vi "Estimate Time.vi"(8 "error in (no error)":errorcluster, 11 "Scheduler in":refnum<class "Scheduler.lvclass">) -> (0 "error out":errorcluster, 3 "Scheduler out":refnum<class "Scheduler.lvclass">)   [LabVIEW 2020, in "Scheduler.lvlib" / "Scheduler.lvclass"]
uses:
  Scheduler.lvclass
  Scheduler.lvclass/Scheduler.ctl
  Run Utilities/Sequence of SBlocks/Sequence of SBlocks.lvclass
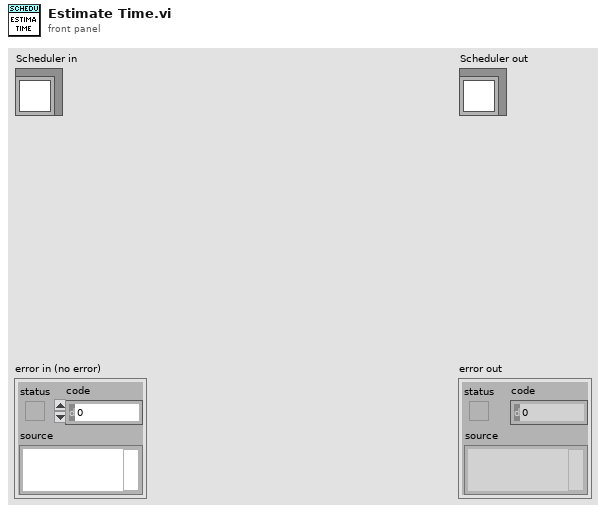
[diagram p1: front panel]
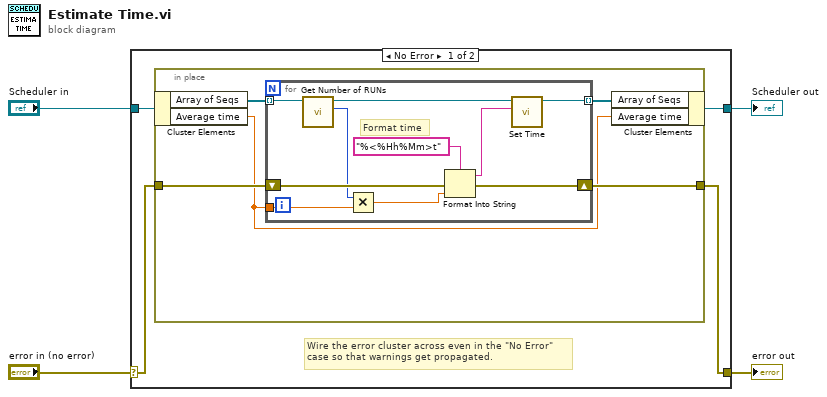
[diagram p0: block diagram]
diagram:
  n1 = case shown="No Error" "error in (no error)" {
    selector: "error in (no error)" -> [w7 w25]
    tunnel: [w6 w25] -> w3
    tunnel: [w5 w24] -> w1
    tunnel: "Scheduler in" -> [w8 w24]
    frame No Error {
      # "Wire the error cluster across even in the \"No Error\"\ncase so that warnings get propagated."
      n2 = in-place {
        in-place-border: w7 -> [w12]
        in-place-border: [w11] -> w6
        n3 = in-place-cluster #1(w8) -> ("Array of Seqs"=w13:refnum<class "Sequence of SBlocks.lvclass">[], "Average time"=w9:dbl)
        n4 = for {
          tunnel: w13 -> [w23] mode=indexing
          shift-right: [w20] -> w11
          shift-left: w12 -> [w21]
          tunnel: w9 -> [w14]
          tunnel: [w16] -> w10 mode=indexing
          # "Format time"
          n5 = call-dynamic "Get Number of RUNs.vi"("Sequence of SBlocks in"=w23) -> ("No of RUNs"=w19:i32, "Sequence of SBlocks out"=w18:refnum<class "Sequence of SBlocks.lvclass">)  [unwired: 8 in, 1 out]
          n6 = Multiply(x=w19, y=w14) -> (x*y=w15:dbl)
          n7 = Format Into String(format string="%<%Hh%Mm>t" ("time format string (%c)"), error in=w21, w15) -> (resulting string=w17:string, error out=w20:errorcluster)  [unwired: 1 in]
          n8 = call-dynamic "Set Time.vi"("Time"=w17, "Sequence of SBlocks in"=w18) -> ("Sequence of SBlocks out"=w16:refnum<class "Sequence of SBlocks.lvclass">)  [unwired: 8 in, 1 out]
        }
        n9 = in-place-cluster #1("Array of Seqs"=w10, "Average time"=w9) -> (w5:refnum<class "Scheduler.lvclass">)
      }
    }
    frame Error {
    }
  }
  "error out" <- w3
  "Scheduler out" <- w1
